vi "eucDist.vi"(1 "y2":dbl=4.0, 2 "x2":dbl=3.0, 3 "y1":dbl, 4 "x1":dbl) -> (0 "d":dbl=5.830951894845301)   [LabVIEW 2017]
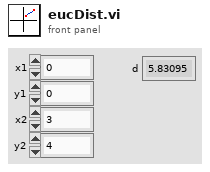
[diagram p1: front panel]
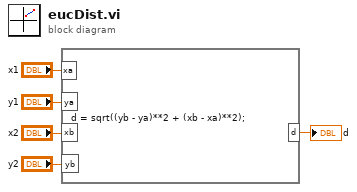
[diagram p0: block diagram]
diagram:
  n1 = formula code="d = sqrt((yb - ya)**2 + (xb - xa)**2);"("xa"="x1", "ya"="y1", "xb"="x2", "yb"="y2") -> ("d"=→"d":dbl)
